vi "calcDist.vi"(0 "X-cord":dbl, 1 "Y-cord":dbl) -> (2 "Distance sideways to pixel":dbl, 3 "Distance to pixel":dbl, 4 "Angle to pixel":dbl)   [LabVIEW 2009, in "ImageAnalysis.lvlib"]
uses:
  ImageAnalysis.lvlib
panel:
  out "x+y":dbl
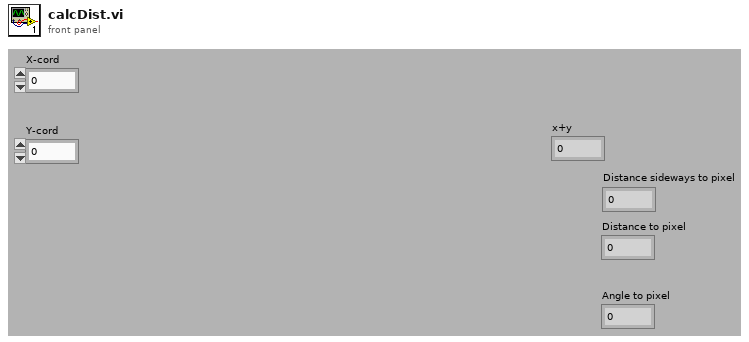
[diagram p1: front panel]
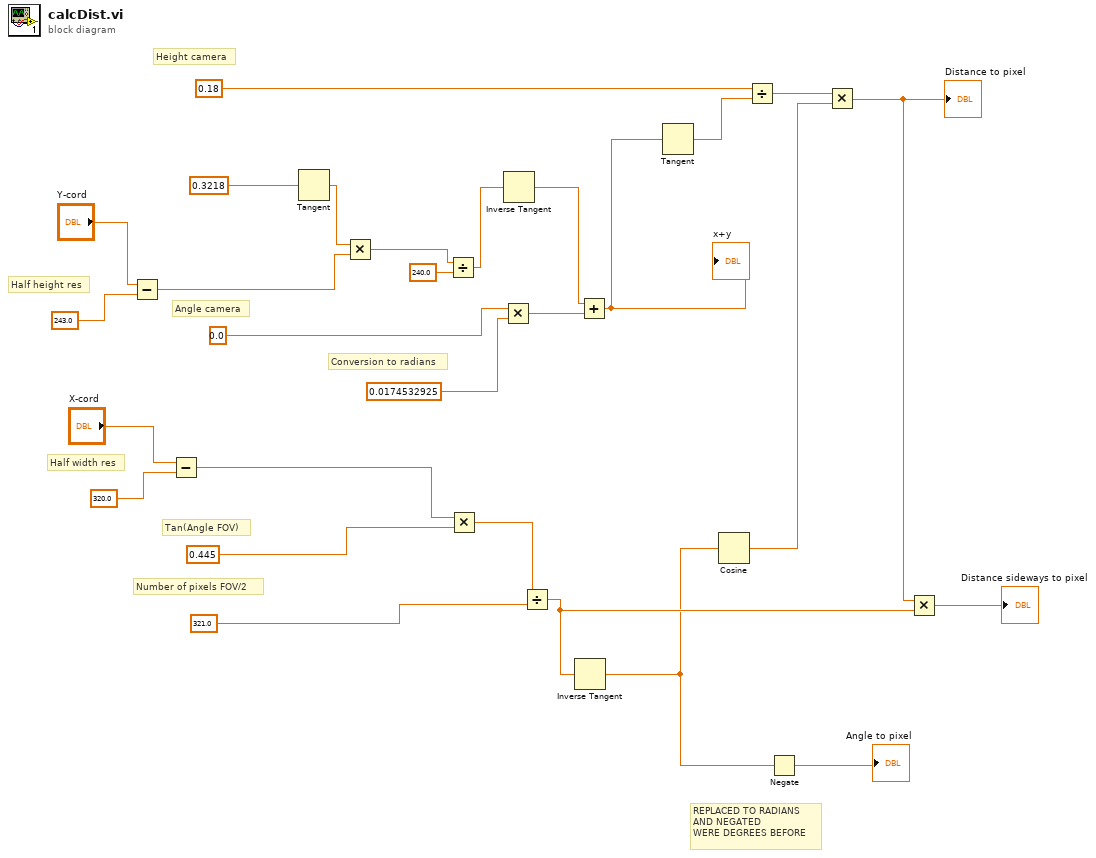
[diagram p0: block diagram]
diagram:
  # "REPLACED TO RADIANS\nAND NEGATED\nWERE DEGREES BEFORE"
  # "Half width res"
  # "Half height res"
  # "Number of pixels FOV/2"
  # "Tan(Angle FOV)"
  # "Conversion to radians"
  # "Angle camera"
  # "Height camera"
  n1 = Subtract(x="Y-cord", y=243.0) -> (x-y=w6:dbl)
  n2 = Subtract(x="X-cord", y=320.0) -> (x-y=w3:dbl)
  n3 = Tangent(1:0.3218 ("x")) -> (0:w24:dbl)
  n4 = Multiply(x=w24, y=w6) -> (x*y=w23:dbl)
  n5 = Divide(x=w23, y=240.0) -> (x/y=w21:dbl)
  n6 = Multiply(x=w3, y=0.445) -> (x*y=w16:dbl)
  n7 = Multiply(x=0.0 ("y"), y=0.0174532925) -> (x*y=w20:dbl)
  n8 = Inverse Tangent(1:w21) -> (0:w19:dbl)
  n9 = Divide(x=w16, y=321.0) -> (x/y=w13:dbl)
  n10 = Inverse Tangent(1:w13) -> (0:w1:dbl)
  n11 = Add(x=w19, y=w20) -> (x+y=w18:dbl)
  "x+y" <- w18
  n12 = Tangent(1:w18) -> (0:w26:dbl)
  n13 = Cosine(x=w1) -> (cos(x)=w10:dbl)
  n14 = Divide(x=0.18, y=w26) -> (x/y=w11:dbl)
  n15 = Negate(x=w1) -> (-x=→"Angle to pixel":dbl)
  n16 = Multiply(x=w11, y=w10) -> (x*y=w9:dbl)
  "Distance to pixel" <- w9
  n17 = Multiply(x=w9, y=w13) -> (x*y=→"Distance sideways to pixel":dbl)
